vi "GetAppFromXRef.vi"(8 "error in (no error)":errorcluster, 11 "XNode Refnum":refnum<vi>) -> (0 "error out":errorcluster, 3 "Owning Application":refnum<vi>)   [LabVIEW 2020, in "NI_XNodeSupport.lvlib"]
uses:
  <vilib>/XNodeSupport/NI_XNodeSupport.lvlib
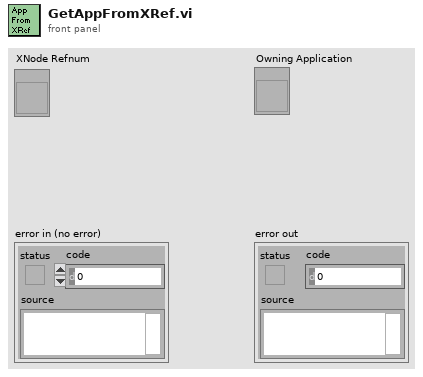
[diagram p1: front panel]
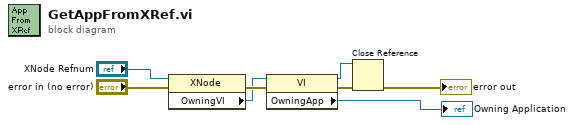
[diagram p0: block diagram]
diagram:
  n1 = property class="XNode"(reference="XNode Refnum", error in="error in (no error)") -> (error out=w7:errorcluster, "OwningVI"=w6:refnum<vi>)  [unwired: 1 out]
  n2 = property class="VI"(reference=w6, error in=w7) -> (reference out=w4:refnum<vi>, error out=w5:errorcluster, "OwningApp"=→"Owning Application":refnum<vi>)
  n3 = Close Reference(reference=w4, error in (no error)=w5) -> (error out=→"error out":errorcluster)
